vi "SendData.vi"(4 "error out 2":errorcluster, 5 "String":string, 6 "byte count":u32, 7 "VISA resource name out 2":refnum<visa-resource-name>) -> (0 "error out":errorcluster, 1 "read buffer":string, 2 "VISA resource name out":refnum<visa-resource-name>, 3 "status_1_OK":i32)   [LabVIEW 2017]
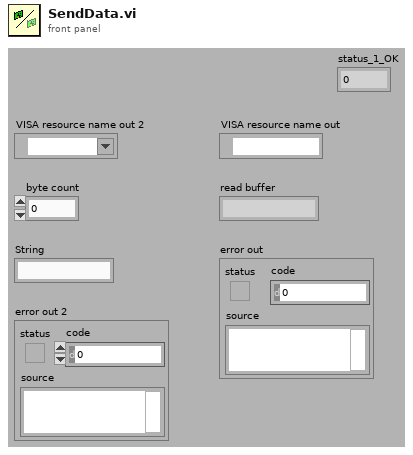
[diagram p1: front panel]
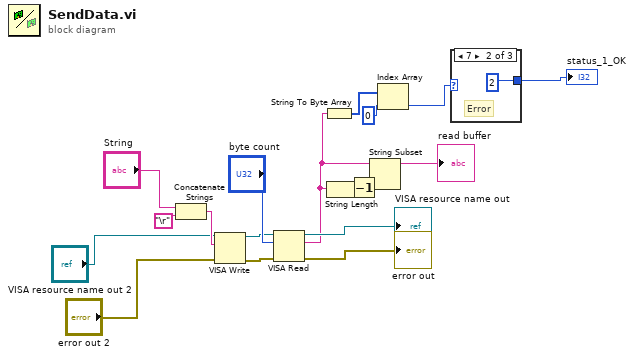
[diagram p0: block diagram]
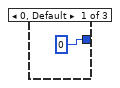
[diagram p2: hidden frame]
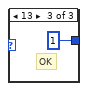
[diagram p3: hidden frame]
diagram:
  n1 = Concatenate Strings("String", "\r") -> (w12:string)
  n2 = VISA Write(VISA resource name="VISA resource name out 2", write buffer=w12, error in (no error)="error out 2") -> (VISA resource name out=w14:refnum<visa-resource-name>, error out=w9:errorcluster)  [unwired: 1 out]
  n3 = VISA Read(VISA resource name=w14, byte count="byte count", error in (no error)=w9) -> (VISA resource name out=→"VISA resource name out":refnum<visa-resource-name>, read buffer=w5:string, error out=→"error out":errorcluster)  [unwired: 1 out]
  n4 = String To Byte Array(string=w5) -> (unsigned byte array=w4:u8[])
  n5 = String Length(string=w5) -> (length=w7:i32)
  n6 = Decrement(x=w7) -> (x-1=w6:i32)
  n7 = String Subset(string=w5, length (rest)=w6) -> (substring=→"read buffer":string)  [unwired: 1 in]
  n8 = Index Array(array=w4, index=0) -> (element=w2:u8)
  n9 = case shown="7" w2 {
    tunnel: [0 ("status") 2 ("status") 1 ("status")] -> w1
    frame 0, Default {
    }
    frame 7 {
      # "Error"
    }
    frame 13 {
      # "OK"
    }
  }
  "status_1_OK" <- w1
